vi "Ex 03-5 - A-Scan + Peaks (Dynamic Range Enhanced).vi"() -> ()   [LabVIEW 2026]
uses:
  <instrlib>/MicroPulse/Public/Data/Datatypes/MP - data formatting.ctl
  <instrlib>/MicroPulse/Public/Data/Datatypes/MP - amplitude reporting mode.ctl
  <instrlib>/MicroPulse/Public/Data/Datatypes/MP - averaging.ctl
  <instrlib>/MicroPulse/Public/Data/Datatypes/MP - transmit parameters.ctl
  <instrlib>/MicroPulse/Public/Data/Datatypes/MP - pulser voltage.ctl
  <instrlib>/MicroPulse/Public/Data/Datatypes/MP - pulse damping.ctl
  <instrlib>/MicroPulse/Public/Data/Datatypes/MP - test parameters.ctl
  <instrlib>/MicroPulse/Public/Data/Datatypes/MP - receive parameters.ctl
  <instrlib>/MicroPulse/Public/Data/Datatypes/MP - display gate.ctl
  <instrlib>/MicroPulse/Public/Data/Datatypes/MP - waveform type.ctl
  <instrlib>/MicroPulse/Public/Data/Datatypes/MP - analogue filter.ctl
  <instrlib>/MicroPulse/Public/Data/Datatypes/MP - frequency filter.ctl
  <instrlib>/MicroPulse/Public/Data/Datatypes/MP - digital filtering.ctl
  <instrlib>/MicroPulse/Public/Data/Datatypes/MP - high pass filter.ctl
  <instrlib>/MicroPulse/Public/Data/Datatypes/MP - low pass filter.ctl
  <instrlib>/MicroPulse/Public/Data/Datatypes/TCP config.ctl
  <instrlib>/MicroPulse/Public/Data/Datatypes/MP - peak settings.ctl
  <instrlib>/MicroPulse/Public/Data/Datatypes/MP - hysteresis level.ctl
  <instrlib>/MicroPulse/Public/Data/Datatypes/MP - sample frequency.ctl
  <instrlib>/MicroPulse/Public/Data/Datatypes/MP - instrument type.ctl
  <instrlib>/MicroPulse/Public/Data/Datatypes/MP - data output format.ctl
  <instrlib>/MicroPulse/Public/Data/Datatypes/MP - DRE gain.ctl
  <instrlib>/MicroPulse/Public/Data/Datatypes/MP - echo gate mode.ctl
  <instrlib>/MicroPulse/MicroPulse_Driver.lvlib
panel:
  in  "DRE Hystresis Delay":u8 max=127
  in  "DRE Gain":T1
  in  "PRF":u16=500 caption="[PRF]" min=1 max=20000 step=100 format="%dHz"
  in  "Data Output Format":T2=enum."16-bit Mode"
  out "Instrument Type":T3
  out "Sample Frequency":T4
  out "peak data":cluster{"Time":dbl[], "Level":u16[]}
  in  "Peak Settings":T5={"Upper Threshold"=10, "Hysteresis"=enum."6dB", "# Peaks In Gate"=8} {"# Peaks In Gate" min=1 max=80; "Upper Threshold" min=10}
  in  "Single Scan":bool
  in  "Stop Streaming":bool
  in  "Start Streaming":bool
  out "Command List":string
  in  "QUIT":bool
  out "running average PRF":dbl format="%0.2f"
  out "A-Scan + Peaks":cluster{"timebase":dbl[], "data":u16[]}[](graph)
  out "live error out":errorcluster
  out "message count":i32
  out "System Messages":string
  in  "TCP config":T7={"Connection ID"=refnum, "IP address"="10.1.1.2", "host port"=1067, "OC timeout"=5000, "Read timeout"=2000, "Write timeout"=100} {"Write timeout" format="%dms"; "Read timeout" format="%dms"; "OC timeout" format="%dms"}
  in  "Receive Parameters":T8={"Display Gate"={"Start"=0.0, "Length"=100.0}, "Delay"=0.0, "Waveform Type"=enum."Rectified Signal", "Gain"=0.0, "Analogue Filtering"={"Bandpass"=enum."No change", "Smoothing"=1}, "Digital Filtering"={"High Pass Filter"=enum."None", "Low Pass Filter"=enum."None"}} {"Delay" format="%#_g us"; "Display Gate"."Length" min=0.0 max=64000.0 step=1.0 format="%#_g us"; "Display Gate"."Start" min=0.0 max=64000.0 step=1.0 format="%#_g us"; "Analogue Filtering"."Smoothing" min=1 max=11 step=1; "Gain" min=-6.0 max=70.0 step=0.25 format="%.2fdB"}
  in  "Test Parameters":T16={"Test No."=1, "Tx Channel"=1, "Rx Channel"=1} {"Rx Channel" min=1 max=1024; "Tx Channel" min=1 max=1024}
  in  "Transmit Parameters":T17={"Pulse Voltage"=enum."50V", "Pulse Shape"={"Damping"=enum."660W", "Width"=250}} {"Pulse Shape"."Width" min=16 max=1010 step=50 format="%.0fns"}
  in  "Data Formatting":T20={"Amplitude Mode"=enum."Ascan + Peaks", "Averaging"=enum."None", "Coupling Level"=0} {"Coupling Level" max=4095 step=1}
  # "Example 03.5 - A-scan + Dynamic Range Enhancement\n\nSet all controls to the required values\nbefore running the VI.\n\nWhile running, test parameters may be changed."
  # "Channels MUST be set BEFORE running"
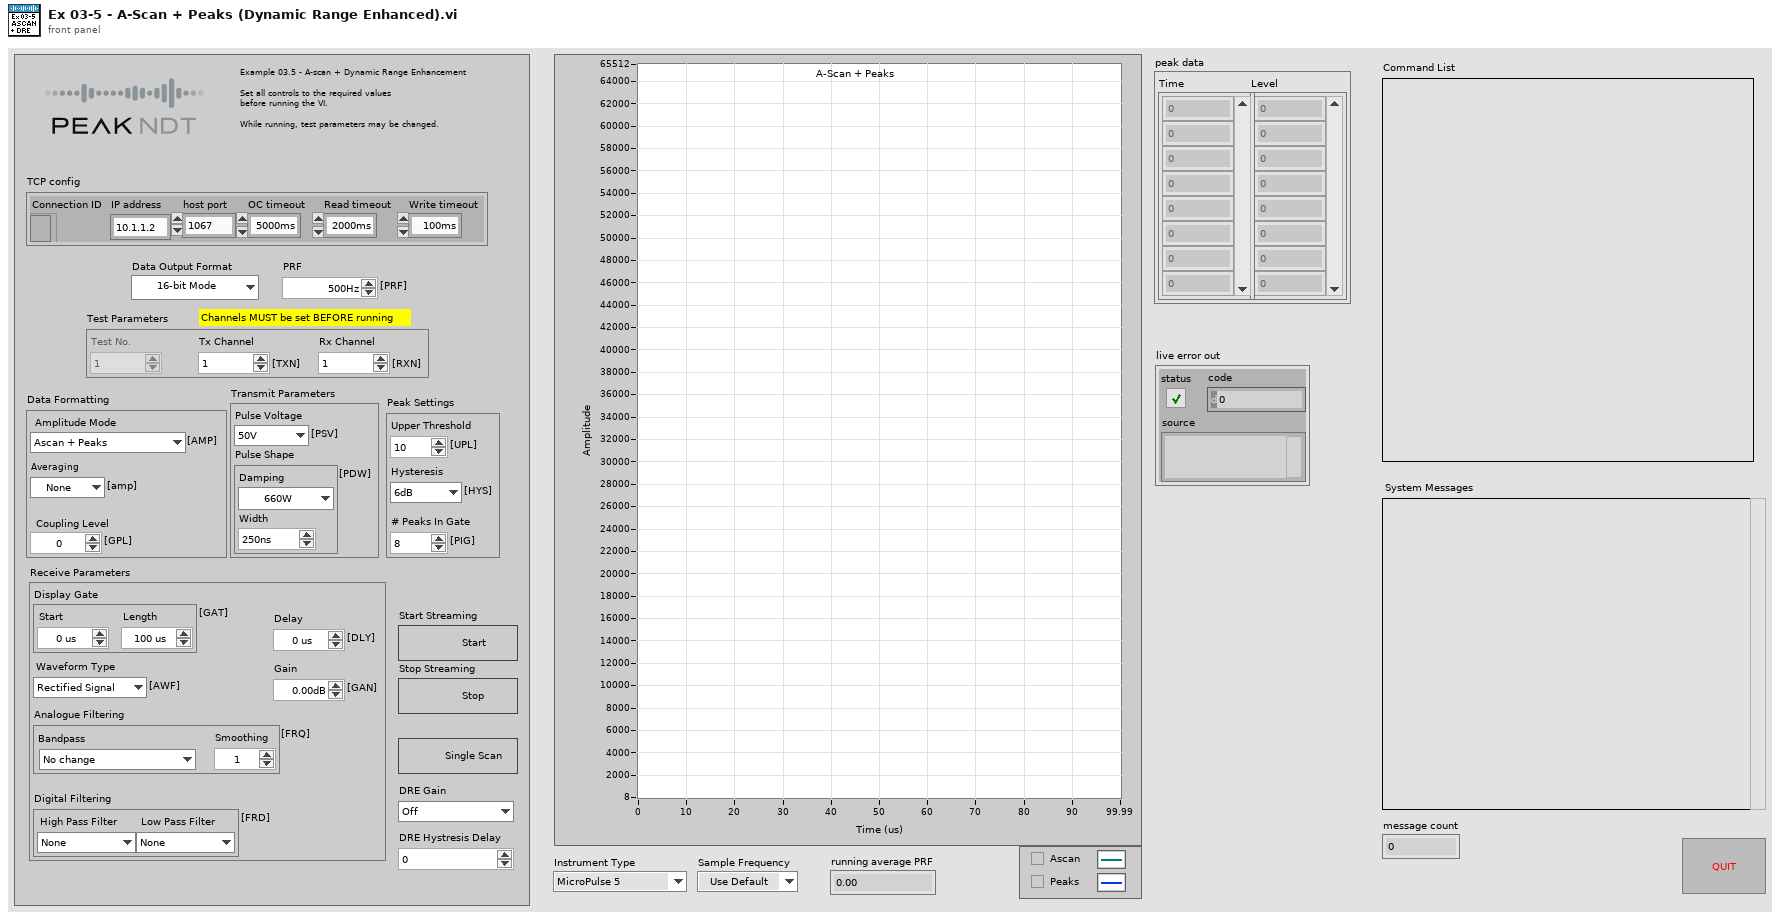
[diagram p1: front panel]
types:
  T1 = typedef "MicroPulse_Driver.lvlib/MP - DRE gain.ctl" = enum16{"Off", "30dB", "36dB", "42dB", "48dB"}
  T2 = typedef "MicroPulse_Driver.lvlib/MP - data output format.ctl" = enum16{"", "8-bit Mode", "10-bit Mode", "12-bit Mode", "16-bit Mode", "8-bit Log Mode", "12-bit Packed Mode"}
  T3 = typedef "MicroPulse_Driver.lvlib/MP - instrument type.ctl" = enum16{"MicroPulse 5", "LT1", "LT2", "LTPA", "MPLT", "MicroPulse 6", "PipeScanner", "<MicroPulse>", "Micropulse 4", "Simulated Data"}
  T4 = typedef "MicroPulse_Driver.lvlib/MP - sample frequency.ctl" = enum16{"Use Default", "200MHz (LT2 only)", "100MHz", "50MHz", "25MHz", "10MHz"}
  T5 = typedef "MicroPulse_Driver.lvlib/MP - peak settings.ctl" = cluster{"Upper Threshold":u16, "Hysteresis":T6, "# Peaks In Gate":u16}
  T6 = typedef "MicroPulse_Driver.lvlib/MP - hysteresis level.ctl" = enum16{"None", "3dB", "6dB", "9dB", "12dB"}
  T7 = typedef "MicroPulse_Driver.lvlib/TCP config.ctl" = cluster{"Connection ID":refnum<k5>, "IP address":string, "host port":u16, "OC timeout":i32, "Read timeout":i32, "Write timeout":i32}
  T8 = typedef "MicroPulse_Driver.lvlib/MP - receive parameters.ctl" = cluster{"Display Gate":T9, "Delay":dbl, "Waveform Type":T10, "Gain":dbl, "Analogue Filtering":T11, "Digital Filtering":T13}
  T9 = typedef "MicroPulse_Driver.lvlib/MP - display gate.ctl" = cluster{"Start":dbl, "Length":dbl}
  T10 = typedef "MicroPulse_Driver.lvlib/MP - waveform type.ctl" = enum16{"Rectified Signal", "RF Signal", "+Half Wave", "-Half Wave"}
  T11 = typedef "MicroPulse_Driver.lvlib/MP - analogue filter.ctl" = cluster{"Bandpass":T12, "Smoothing":u16}
  T12 = typedef "MicroPulse_Driver.lvlib/MP - frequency filter.ctl" = enum16{"No change", "1MHz Bandpass", "2MHz Bandpass", "4MHz Bandpass", "5MHz Bandpass", "10MHz Bandpass", "2.5-18MHz Broadband", "0.75-12MHz  Broadband", "0.5MHz Bandpass", "5MHz 2nd Order TOFD", "10MHz 2nd Order TOFD", "3.0-25MHz Broadband", "3.0-30MHz Broadband"}
  T13 = typedef "MicroPulse_Driver.lvlib/MP - digital filtering.ctl" = cluster{"High Pass Filter":T14, "Low Pass Filter":T15}
  T14 = typedef "MicroPulse_Driver.lvlib/MP - high pass filter.ctl" = enum16{"None", "0.7MHz", "1.5MHz", "4.0MHz", "7.5MHz", "10.0MHz", "User Defined"}
  T15 = typedef "MicroPulse_Driver.lvlib/MP - low pass filter.ctl" = enum16{"None", "1.8MHz", "3.0MHz", "6.0MHz", "8.0MHz", "12.0MHz", "User Defined"}
  T16 = typedef "MicroPulse_Driver.lvlib/MP - test parameters.ctl" = cluster{"Test No.":u32, "Tx Channel":u32, "Rx Channel":u32}
  T17 = typedef "MicroPulse_Driver.lvlib/MP - transmit parameters.ctl" = cluster{"Pulse Voltage":T18, "Pulse Shape":cluster{"Damping":T19, "Width":u32}}
  T18 = typedef "MicroPulse_Driver.lvlib/MP - pulser voltage.ctl" = enum16{"50V", "100V", "150V", "200V", "250V", "300V"}
  T19 = typedef "MicroPulse_Driver.lvlib/MP - pulse damping.ctl" = enum16{"660W", "458W", "220W", "149W", "102W", "82W", "63W", "51W"}
  T20 = typedef "MicroPulse_Driver.lvlib/MP - data formatting.ctl" = cluster{"Amplitude Mode":T21, "Averaging":T22, "Coupling Level":u32}
  T21 = typedef "MicroPulse_Driver.lvlib/MP - amplitude reporting mode.ctl" = enum16{"1st Peak in gate", "Maximum Peak in gate", "All Peaks", "Ascan Data", "1st Threshold Crossing Peak", "Ascan + Peaks", "All Peaks for Multigate", "Peaks + Ascan for Multigate", "Peaks + P_Ascan for Multigate", "Full Matrix Capture"}
  T22 = typedef "MicroPulse_Driver.lvlib/MP - averaging.ctl" = enum16{"None", "2", "4", "8", "16", "32", "64", "128", "256"}
  T23 = typedef "MicroPulse_Driver.lvlib/MP - echo gate mode.ctl" = enum16{"Echo Trigger OFF", "Echo Gate Display Mode", "Echo Trigger ON", "Multi Gate or FMC Mode", "Reserved", "PA - Echo Trigger ON"}
  T24 = typedef "MicroPulse_Driver.lvlib/MP-Registry Data-Cluster.ctl" = cluster{"Instrument Type":T3, "Serial #":u64, "Sample Frequency":T4, "dt (us)":dbl, "DOF":T2, "Material Velocity":dbl, "Asynch Reads":T25, "NUM of Tests":u32, "System Details":T26, "Gates":T28[], "Encoders":T32[], "CMD LUT":variant, "Command List":string}
  T25 = typedef "MicroPulse_Driver.lvlib/MP - asynch read mode.ctl" = enum16{"Disabled", "Enabled"}
  T26 = typedef "MicroPulse_Driver.lvlib/MP - general system status.ctl" = cluster{"System Type":T3, "Serial No.":u64, "Channels":cluster{"Conv":u8, "PA":u16, "Extra":u32}, "Sample Frequency":cluster{"Default":u8, "Actual":u8}, "Software Versions":string, "Data Output Format":cluster{"Default":T2, "Actual":T2}, "Temperatures":cluster{"System":u8, "Processor":u8, "Slave Sys":u8, "Slave Proc":u8}, "Tx Buffer Size":u32, "System Error":string, "No. of Cards":u8, "DAC Gain":i16, "Uptimes":cluster{"since Power":u32, "since RSTS":u32, "since SRST":u32}, "Voltages":cluster{"Nominal":dbl, "Measured":dbl, "Difference":dbl}[], "Interface Cards":T27[]}
  T27 = typedef "MicroPulse_Driver.lvlib/MP - interface card status.ctl" = cluster{"Status":u8, "Map":u8, "Board - T":u8, "FPGA - T":u8, "PAIF Status":string, "Version":string}
  T28 = typedef "MicroPulse_Driver.lvlib/MP - Registry Gates.ctl" = cluster{"Display Gate":T9, "ETM Mode":T23, "Echo Gate":T29, "Insp Gates":T30[]}
  T29 = typedef "MicroPulse_Driver.lvlib/MP - echo gate parameters.ctl" = cluster{"Start (us)":dbl, "Length (us)":dbl, "Threshold":u16, "Colour":u32}
  T30 = typedef "MicroPulse_Driver.lvlib/MP - multigate inspection gate parameters.ctl" = cluster{"Start (us)":dbl, "Length (us)":dbl, "Threshold":u16, "Enabled?":bool, "Max # Peaks":u16, "Hysteresis":T6, "Mode":T31, "Inverted?":bool, "Colour ":u32}
  T31 = typedef "MicroPulse_Driver.lvlib/MP - multigate mode.ctl" = enum16{"1st Peak in Gate", "Largest Peak In Gate", "All Peaks In Gate", "1st Threshold Crossing"}
  T32 = typedef "MicroPulse_Driver.lvlib/MP - encoder settings.ctl" = cluster{"Encoder Type":T33, "Counts/mm":u32, "Enable Termination?":bool, "Multiplier":u32, "Backlash Period (s)":dbl, "Encoder Filter":u32}
  T33 = typedef "MicroPulse_Driver.lvlib/MP - encoder type.ctl" = enum16{"Quadrature", "Step/Direction"}
  T34 = typedef "MicroPulse_Driver.lvlib/MP - scan data info.ctl" = cluster{"Message Header":u16, "Error Message":u16, "Test No.":u32, "Channel No.":u8, "Sweep No.":u32, "Gate No.":u32, "DOF":T2, "retain data":T35, "scan data":u16[], "scan length":i32, "scan index":i32, "peak data":cluster{"timebase":u16[], "data":u16[]}, "#peaks":i32, "PRF":dbl, "IP":cluster{"Axis No.":u8, "Location":u32, "MIP location":u32, "MIP?":bool}, "echo range":u16, "ETG":bool, "CAL 0 complete":bool, "Axis Positions":T36}
  T35 = typedef "MicroPulse_Driver.lvlib/MP - retain scan.ctl" = enum16{"None", "Ascan", "Peaks"}
  T36 = typedef "MicroPulse_Driver.lvlib/MP - axis positions (LLC).ctl" = cluster{"Axis 1":u32, "Axis 2":u32, "Axis 3":u32, "Axis 4":u32, "Status":u8}
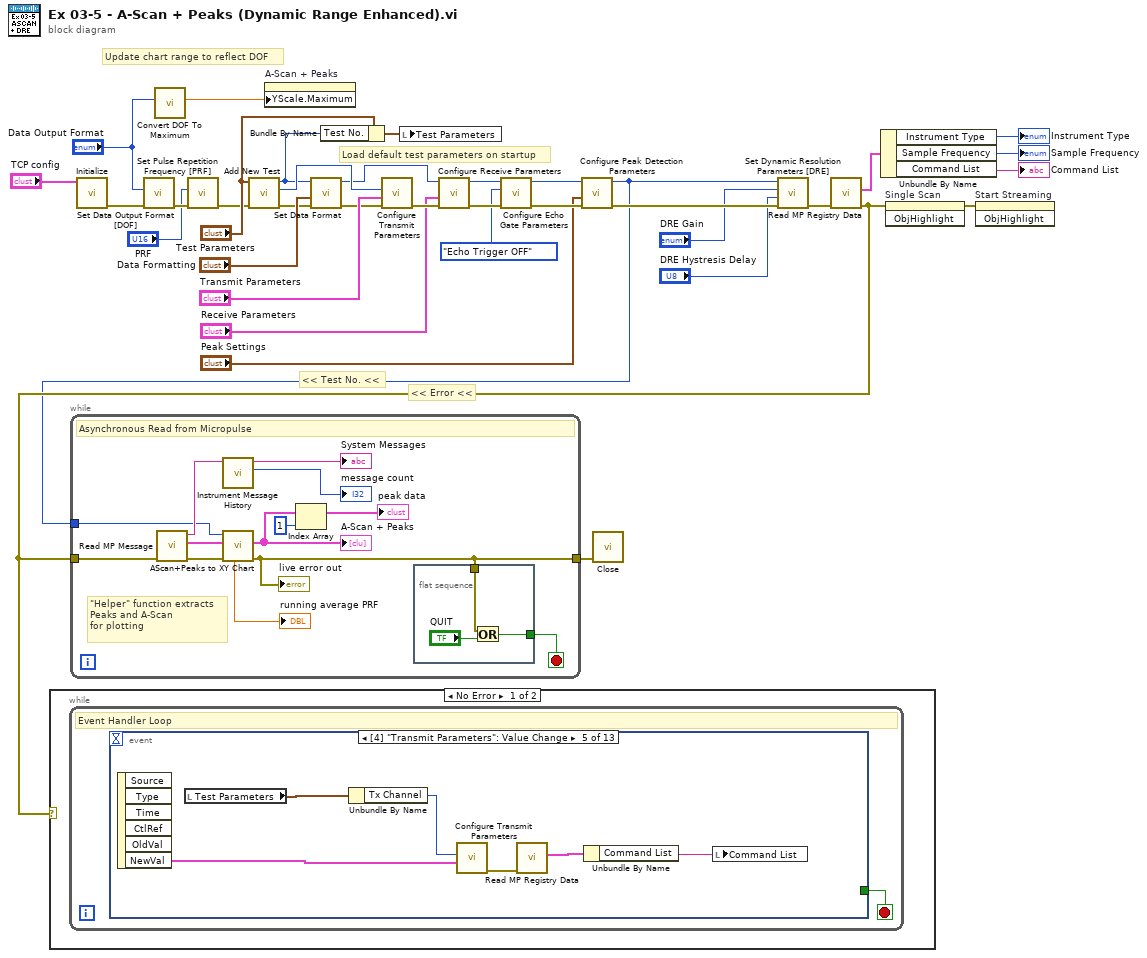
[diagram p0: block diagram]
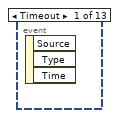
[diagram p2: hidden frame]
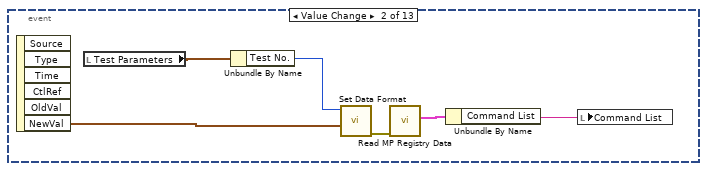
[diagram p3: hidden frame]
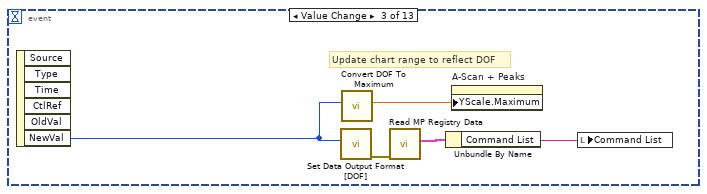
[diagram p4: hidden frame]
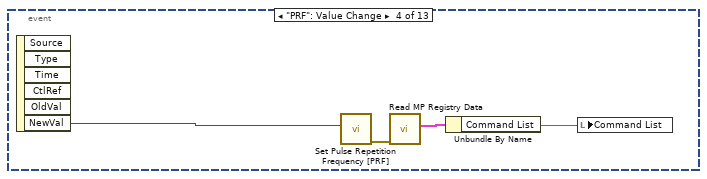
[diagram p5: hidden frame]
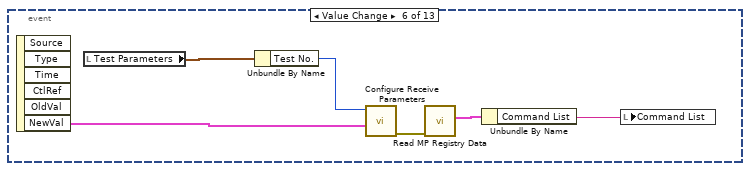
[diagram p6: hidden frame]
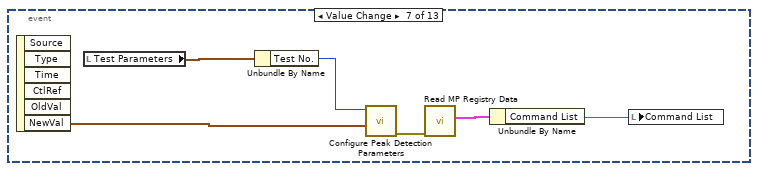
[diagram p7: hidden frame]
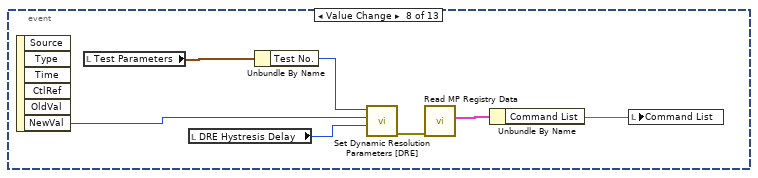
[diagram p8: hidden frame]
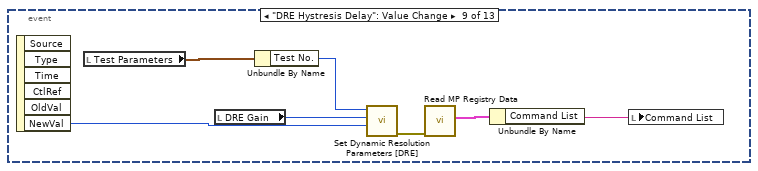
[diagram p9: hidden frame]
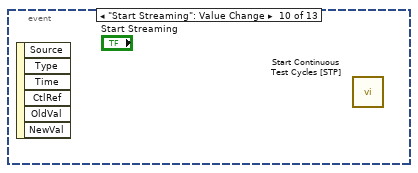
[diagram p10: hidden frame]
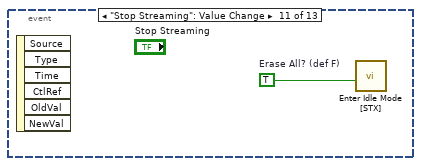
[diagram p11: hidden frame]
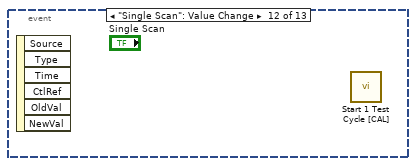
[diagram p12: hidden frame]
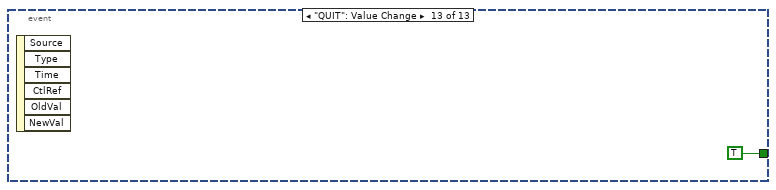
[diagram p13: hidden frame]
diagram:
  # "Update chart range to reflect DOF"
  # "<< Error <<"
  # "<< Test No. <<"
  # "Load default test parameters on startup"
  n1 = call <instrlib>:"Initialize.vi"("TCP config"="TCP config") -> ("error out"=w27:errorcluster)  [unwired: 9 in, 1 out]
  n2 = call <instrlib>:"Set Data Output Format [DOF].vi"("error in (no error)"=w27, "Mode"="Data Output Format") -> ("error out"=w10:errorcluster)  [unwired: 8 in, 1 out]
  n3 = call <instrlib>:"Convert DOF To Maximum.vi"("Data Output Format"="Data Output Format") -> ("Data Maximum"=w7:dbl)  [unwired: 10 in]
  n4 = call <instrlib>:"Set Pulse Repetition Frequency [PRF].vi"("error in (no error)"=w10, "Frequency (Hz)"="PRF") -> ("error out"=w9:errorcluster)  [unwired: 8 in, 1 out]
  n5 = call <instrlib>:"Add New Test.vi"("error in (no error)"=w9, "Test Parameters"="Test Parameters") -> ("error out"=w26:errorcluster, "Tx Channel out"=w25:u32, "Test No. out"=w12:u32)  [unwired: 6 in, 1 out]
  n6 = property on="A-Scan + Peaks" class="XYGraph (strict)"("YScale.Maximum"=w7) -> ()  [unwired: 2 in, 2 out]
  n7 = call <instrlib>:"Set Data Format.vi"("error in (no error)"=w26, "Data Formatting"="Data Formatting", "Test No."=w12) -> ("error out"=w32:errorcluster, "Test No. out"=w24:u32)  [unwired: 6 in, 1 out]
  n8 = Bundle By Name(cluster="Test Parameters", "Test No."=w12) -> (w11:T16)
  n9 = call <instrlib>:"Configure Transmit Parameters.vi"("error in (no error)"=w32, "Transmit Parameters"="Transmit Parameters", "Tx Channel"=w25) -> ("error out"=w33:errorcluster)  [unwired: 7 in, 1 out]
  n10 = local write "Test Parameters"(w11) -> ()
  n11 = call <instrlib>:"Configure Receive Parameters.vi"("error in (no error)"=w33, "Receive Parameters"="Receive Parameters", "Test No."=w24) -> ("error out"=w31:errorcluster, "Test No. out"=w23:u32)  [unwired: 6 in, 1 out]
  n12 = call <instrlib>:"Configure Echo Gate Parameters.vi"("error in (no error)"=w31, "Echo Trigger Mode"=MP_-_echo_gate_mode."Echo Trigger OFF" ("ETM Mode"), "Test Number"=w23) -> ("error out"=w21:errorcluster, "Test Number Out"=w22:u32)  [unwired: 6 in, 1 out]
  n13 = call <instrlib>:"Configure Peak Detection Parameters.vi"("error in (no error)"=w21, "Peak Settings"="Peak Settings", "Test Number"=w22) -> ("error out"=w5:errorcluster, "Test Number Out"=w1:u32)  [unwired: 6 in, 1 out]
  n14 = call <instrlib>:"Set Dynamic Resolution Parameters [DRE].vi"("error in (no error)"=w5, "DRE Hysteresis Delay"="DRE Hystresis Delay", "DRE Gain"="DRE Gain", "Test No."=w1) -> ("error out"=w4:errorcluster)  [unwired: 6 in, 1 out]
  n15 = call <instrlib>:"Read MP Registry Data.vi"("error in (no error)"=w4) -> ("error out"=w17:errorcluster, "Micropulse Data"=w19:T24)  [unwired: 7 in, 2 out]
  n16 = case shown="No Error" w17 {
    frame No Error {
      n17 = while {
        stop <- w37 stop-if-true
        # "Event Handler Loop"
        n18 = event shown="[4] \"Transmit Parameters\": Value Change" {
          selector: _ -> [_ _ _ _ _ _ _ _ _ _ _ _ _]
          dyn-events: _ -> [_ _ _ _ _ _ _ _ _ _ _ _ _]
          timeout: _ -> [_ _ _ _ _ _ _ _ _ _ _ _ _]
          tunnel: [_ _ _ _ _ _ _ _ _ _ _ _ TRUE ("stop")] -> w37
          event Timeout {
            n19 = event-data() -> ()  [unwired: 1 in, 3 out]
          }
          event Value Change {
            n20 = event-data() -> ("NewVal"=w43:T20)  [unwired: 1 in, 5 out]
            n21 = local read "Test Parameters"() -> (w42:T16)
            n22 = Unbundle By Name(w42) -> ("Test No."=w41:u32)
            n23 = call <instrlib>:"Set Data Format.vi"("Data Formatting"=w43, "Test No."=w41) -> ("error out"=w39:errorcluster)  [unwired: 7 in, 2 out]
            n24 = call <instrlib>:"Read MP Registry Data.vi"("error in (no error)"=w39) -> ("Micropulse Data"=w40:T24)  [unwired: 7 in, 3 out]
            n25 = Unbundle By Name(w40) -> ("Command List"=w38:string)
            n26 = local write "Command List"(w38) -> ()
          }
          event Value Change {
            # "Update chart range to reflect DOF"
            n27 = event-data() -> ("NewVal"=w44:T2)  [unwired: 1 in, 5 out]
            n28 = call <instrlib>:"Set Data Output Format [DOF].vi"("Mode"=w44) -> ("error out"=w47:errorcluster)  [unwired: 9 in, 1 out]
            n29 = call <instrlib>:"Convert DOF To Maximum.vi"("Data Output Format"=w44) -> ("Data Maximum"=w45:dbl)  [unwired: 10 in]
            n30 = call <instrlib>:"Read MP Registry Data.vi"("error in (no error)"=w47) -> ("Micropulse Data"=w48:T24)  [unwired: 7 in, 3 out]
            n31 = Unbundle By Name(w48) -> ("Command List"=w46:string)
            n32 = property on="A-Scan + Peaks" class="XYGraph (strict)"("YScale.Maximum"=w45) -> ()  [unwired: 2 in, 2 out]
            n33 = local write "Command List"(w46) -> ()
          }
          event "PRF": Value Change {
            n34 = event-data() -> ("NewVal"=w49:u16)  [unwired: 1 in, 5 out]
            n35 = call <instrlib>:"Set Pulse Repetition Frequency [PRF].vi"("Frequency (Hz)"=w49) -> ("error out"=w51:errorcluster)  [unwired: 9 in, 1 out]
            n36 = call <instrlib>:"Read MP Registry Data.vi"("error in (no error)"=w51) -> ("Micropulse Data"=w52:T24)  [unwired: 7 in, 3 out]
            n37 = Unbundle By Name(w52) -> ("Command List"=w50:string)
            n38 = local write "Command List"(w50) -> ()
          }
          event Value Change {
            n39 = event-data() -> ("NewVal"=w57:T17)  [unwired: 1 in, 5 out]
            n40 = local read "Test Parameters"() -> (w58:T16)
            n41 = Unbundle By Name(w58) -> ("Tx Channel"=w56:u32)
            n42 = call <instrlib>:"Configure Transmit Parameters.vi"("Transmit Parameters"=w57, "Tx Channel"=w56) -> ("error out"=w54:errorcluster)  [unwired: 8 in, 1 out]
            n43 = call <instrlib>:"Read MP Registry Data.vi"("error in (no error)"=w54) -> ("Micropulse Data"=w55:T24)  [unwired: 7 in, 3 out]
            n44 = Unbundle By Name(w55) -> ("Command List"=w53:string)
            n45 = local write "Command List"(w53) -> ()
          }
          event Value Change {
            n46 = event-data() -> ("NewVal"=w60:T8)  [unwired: 1 in, 5 out]
            n47 = local read "Test Parameters"() -> (w64:T16)
            n48 = Unbundle By Name(w64) -> ("Test No."=w63:u32)
            n49 = call <instrlib>:"Configure Receive Parameters.vi"("Receive Parameters"=w60, "Test No."=w63) -> ("error out"=w62:errorcluster)  [unwired: 7 in, 2 out]
            n50 = call <instrlib>:"Read MP Registry Data.vi"("error in (no error)"=w62) -> ("Micropulse Data"=w61:T24)  [unwired: 7 in, 3 out]
            n51 = Unbundle By Name(w61) -> ("Command List"=w59:string)
            n52 = local write "Command List"(w59) -> ()
          }
          event Value Change {
            n53 = event-data() -> ("NewVal"=w66:T5)  [unwired: 1 in, 5 out]
            n54 = local read "Test Parameters"() -> (w70:T16)
            n55 = Unbundle By Name(w70) -> ("Test No."=w69:u32)
            n56 = call <instrlib>:"Configure Peak Detection Parameters.vi"("Peak Settings"=w66, "Test Number"=w69) -> ("error out"=w68:errorcluster)  [unwired: 7 in, 2 out]
            n57 = call <instrlib>:"Read MP Registry Data.vi"("error in (no error)"=w68) -> ("Micropulse Data"=w67:T24)  [unwired: 7 in, 3 out]
            n58 = Unbundle By Name(w67) -> ("Command List"=w65:string)
            n59 = local write "Command List"(w65) -> ()
          }
          event Value Change {
            n60 = event-data() -> ("NewVal"=w72:T1)  [unwired: 1 in, 5 out]
            n61 = local read "Test Parameters"() -> (w77:T16)
            n62 = local read "DRE Hystresis Delay"() -> (w71:u8)
            n63 = Unbundle By Name(w77) -> ("Test No."=w73:u32)
            n64 = call <instrlib>:"Set Dynamic Resolution Parameters [DRE].vi"("DRE Hysteresis Delay"=w71, "DRE Gain"=w72, "Test No."=w73) -> ("error out"=w74:errorcluster)  [unwired: 7 in, 1 out]
            n65 = call <instrlib>:"Read MP Registry Data.vi"("error in (no error)"=w74) -> ("Micropulse Data"=w76:T24)  [unwired: 7 in, 3 out]
            n66 = Unbundle By Name(w76) -> ("Command List"=w75:string)
            n67 = local write "Command List"(w75) -> ()
          }
          event "DRE Hystresis Delay": Value Change {
            n68 = event-data() -> ("NewVal"=w78:u8)  [unwired: 1 in, 5 out]
            n69 = local read "Test Parameters"() -> (w84:T16)
            n70 = local read "DRE Gain"() -> (w79:T1)
            n71 = Unbundle By Name(w84) -> ("Test No."=w80:u32)
            n72 = call <instrlib>:"Set Dynamic Resolution Parameters [DRE].vi"("DRE Hysteresis Delay"=w78, "DRE Gain"=w79, "Test No."=w80) -> ("error out"=w81:errorcluster)  [unwired: 7 in, 1 out]
            n73 = call <instrlib>:"Read MP Registry Data.vi"("error in (no error)"=w81) -> ("Micropulse Data"=w83:T24)  [unwired: 7 in, 3 out]
            n74 = Unbundle By Name(w83) -> ("Command List"=w82:string)
            n75 = local write "Command List"(w82) -> ()
          }
          event "Start Streaming": Value Change {
            n76 = event-data() -> ()  [unwired: 1 in, 6 out]
            n77 = call <instrlib>:"Start Continuous Test Cycles [STP].vi"() -> ()  [unwired: 10 in, 2 out]
          }
          event "Stop Streaming": Value Change {
            w85 = TRUE  # Erase All? (def F)
            n78 = event-data() -> ()  [unwired: 1 in, 6 out]
            n79 = call <instrlib>:"Enter Idle Mode [STX].vi"("Erase All? (def T)"=w85) -> ()  [unwired: 9 in, 2 out]
          }
          event "Single Scan": Value Change {
            n80 = event-data() -> ()  [unwired: 1 in, 6 out]
            n81 = call <instrlib>:"Start 1 Test Cycle [CAL].vi"() -> ()  [unwired: 10 in, 2 out]
          }
          event "QUIT": Value Change {
            n82 = event-data() -> ()  [unwired: 1 in, 6 out]
          }
        }
      }
    }
    frame Error {
    }
  }
  n83 = while {
    tunnel: [w88] -> w30
    tunnel: w17 -> [w95]
    tunnel: w1 -> [w93]
    stop <- w98 stop-if-true
    # "\"Helper\" function extracts\nPeaks and A-Scan\nfor plotting"
    # "Asynchronous Read from Micropulse"
    n84 = call <instrlib>:"Read MP Message.vi"("error in (no error)"=w95) -> ("error out"=w94:errorcluster, "scan data info"=w92:T34, "Instrument Message"=w97:string)  [unwired: 6 in, 2 out]
    n85 = call <instrlib>:"Instrument Message History.vi"("Instrument Message"=w97) -> ("Message Count"=→"message count":i32, "Message History out"=→"System Messages":string)  [unwired: 9 in]
    n86 = call <instrlib>:"AScan+Peaks to XY Chart.vi"("error in (no error)"=w94, "scan data info"=w92, "Test No."=w93) -> ("error out"=w88:errorcluster, "AScan+Peaks"=w91:cluster{"timebase":dbl[], "data":u16[]}[], "Running Average PRF"=→"running average PRF":dbl)  [unwired: 3 in, 3 out]
    "A-Scan + Peaks" <- w91
    "live error out" <- w88
    n87 = Index Array(array=w91, index=1) -> (element=→"peak data":cluster{"timebase":dbl[], "data":u16[]})
    n88 = flat-sequence {
      tunnel: [w101] -> w98
      tunnel: w88 -> [w100]
      frame #0 {
        n89 = Or(x=w100, y="QUIT") -> (x .or. y?=w101:bool)
      }
    }
  }
  n90 = call <instrlib>:"Close.vi"("error in (no error)"=w30) -> ()  [unwired: 9 in, 2 out]
  n91 = Unbundle By Name(w19) -> ("Instrument Type"=→"Instrument Type":T3, "Sample Frequency"=→"Sample Frequency":T4, "Command List"=→"Command List":string)
  n92 = invoke on="Single Scan" class="Bool" method="ObjHighlight"(error in=w17) -> (error out=w16:errorcluster)  [unwired: 2 in, 2 out]
  n93 = invoke on="Start Streaming" class="Bool" method="ObjHighlight"(error in=w16) -> ()  [unwired: 2 in, 3 out]
